vi "get_radius_array.vi"(8 "error in (no error)":errorcluster, 11 "TrajectoryDL110420DoubleCircle in":refnum<class "TrajectoryDL110420DoubleCircle.lvclass">) -> (0 "error out":errorcluster, 2 "radius array":dbl[unit][](array[numeric]), 3 "TrajectoryDL110420DoubleCircle out":refnum<class "TrajectoryDL110420DoubleCircle.lvclass">)   [LabVIEW 2010, in "TrajectoryDL110420DoubleCircle.lvclass"]
uses:
  TrajectoryDL110420DoubleCircle.lvclass
  TrajectoryDL110420DoubleCircle.lvclass/TrajectoryDL110420DoubleCircle.ctl
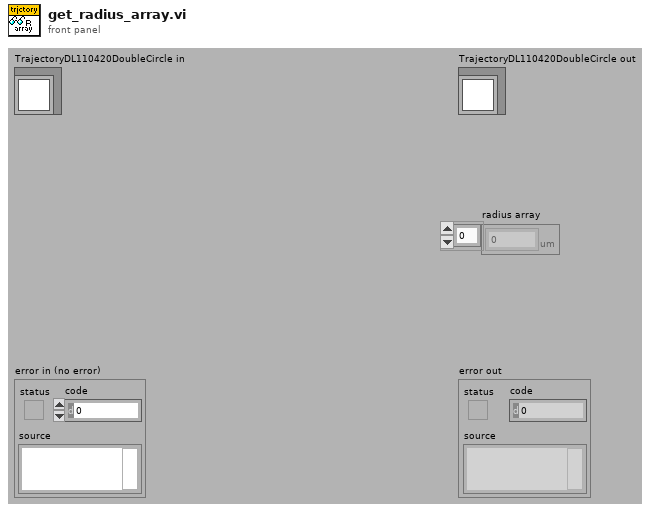
[diagram p1: front panel]
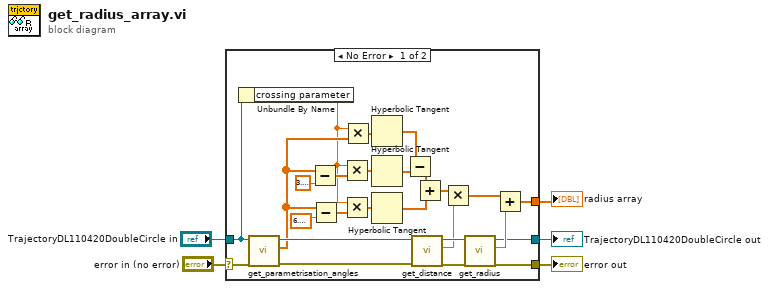
[diagram p0: block diagram]
diagram:
  n1 = case shown="No Error" "error in (no error)" {
    selector: "error in (no error)" -> [w29 w33]
    tunnel: [w26 w33] -> w4
    tunnel: [w6 w32] -> w2
    tunnel: "TrajectoryDL110420DoubleCircle in" -> [w16 w32]
    tunnel: [w7 _] -> w1
    frame No Error {
      n2 = Unbundle By Name(w16) -> ("crossing parameter"=w13:dbl)
      n3 = call-dynamic "get_parametrisation_angles.vi"("error in (no error)"=w29, "TrajectoryDL110420DoubleCircle in"=w16) -> ("error out"=w30:errorcluster, "angles"=w19:dbl[], "TrajectoryDL110420DoubleCircle out"=w28:refnum<class "TrajectoryDL110420DoubleCircle.lvclass">)  [unwired: 7 in]
      n4 = Subtract(x=w19, y=3.141592653589793) -> (x-y=w15:dbl[])
      n5 = Subtract(x=w19, y=6.283185307179586) -> (x-y=w14:dbl[])
      n6 = Multiply(x=w13, y=w15) -> (x*y=w20:dbl[])
      n7 = Multiply(x=w13, y=w14) -> (x*y=w17:dbl[])
      n8 = Multiply(x=w13, y=w19) -> (x*y=w31:dbl[])
      n9 = Hyperbolic Tangent(1:w31) -> (0:w12:dbl[])
      n10 = Hyperbolic Tangent(1:w20) -> (0:w11:dbl[])
      n11 = Hyperbolic Tangent(1:w17) -> (0:w9:dbl[])
      n12 = Subtract(x=w12, y=w11) -> (x-y=w10:dbl[])
      n13 = call-dynamic "get_distance.vi"("error in (no error)"=w30, "TrajectoryDL110420DoubleCircle in"=w28) -> ("error out"=w27:errorcluster, "distance"=w21:dbl[unit], "TrajectoryDL110420DoubleCircle out"=w25:refnum<class "TrajectoryDL110420DoubleCircle.lvclass">)  [unwired: 7 in]
      n14 = Add(x=w10, y=w9) -> (x+y=w8:dbl[])
      n15 = Multiply(x=w8, y=w21) -> (x*y=w24:dbl[unit][])
      n16 = call-dynamic "get_radius.vi"("error in (no error)"=w27, "TrajectoryDL110420DoubleCircle in"=w25) -> ("error out"=w26:errorcluster, "radius"=w23:dbl[unit], "TrajectoryDL110420DoubleCircle out"=w6:refnum<class "TrajectoryDL110420DoubleCircle.lvclass">)  [unwired: 7 in]
      n17 = Add(x=w24, y=w23) -> (x+y=w7:dbl[unit][])
    }
    frame Error {
    }
  }
  "error out" <- w4
  "TrajectoryDL110420DoubleCircle out" <- w2
  "radius array" <- w1
